vi "display AP status.vi"(7 "in or out display Refnum":refnum<vi>, 8 "error in":errorcluster={"status"=FALSE, "code"=-1950679034, "source"="Shared Variable in Large VAC READBACKS.vi<APPEND>\nThis error or warning occurred while reading the following Shared Variable:\n\\\\My Computer\\lowendshmc\\digital outputs\n\\\\192.168.1.200\\lowendshmc\\digital outputs"}, 9 "Aperture Status":T1, 10 "device control Refnum":refnum<vi>, 11 "use color control":bool) -> (0 "error out":errorcluster={"status"=FALSE, "code"=-1950679034, "source"="Shared Variable in Large VAC READBACKS.vi<APPEND>\nThis error or warning occurred while reading the following Shared Variable:\n\\\\My Computer\\lowendshmc\\digital outputs\n\\\\192.168.1.200\\lowendshmc\\digital outputs"})   [LabVIEW 2016, in "sub-VIs.lvlib"]
doc: "controls the display of if a cup or apt. is in the beamline"
uses:
  sub-VIs/sub-VIs.lvlib
  controls/Aperture states.ctl
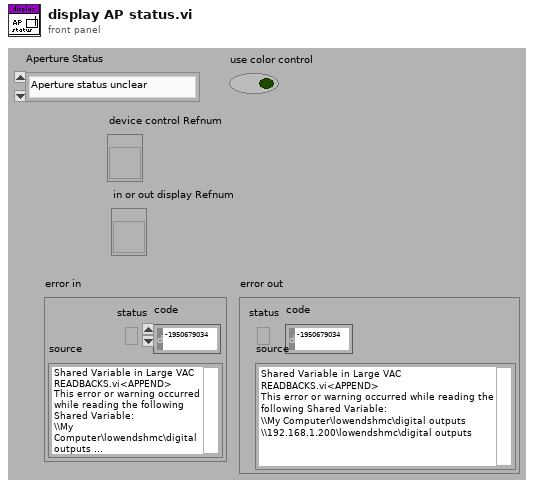
[diagram p1: front panel]
types:
  T1 = typedef "Aperture states.ctl" = enum16{"Aperture status unclear", "Aperture in", "Aperture out"}
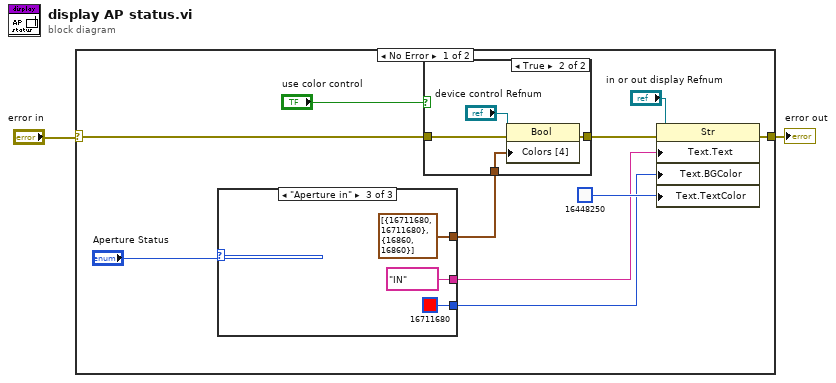
[diagram p0: block diagram]
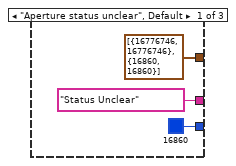
[diagram p3: hidden frame]
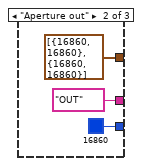
[diagram p4: hidden frame]
diagram:
  n1 = case shown="No Error" "error in" {
    selector: "error in" -> [w5 w27]
    tunnel: [w6 w27] -> w2
    frame No Error {
      n2 = case shown="\"Aperture in\"" "Aperture Status" {
        tunnel: ["Status Unclear" ("Text.Text") "OUT" ("Text.Text") "IN" ("Text.Text")] -> w9
        tunnel: [u32 16860 u32 16860 u32 16711680] -> w10
        tunnel: [cluster{u32, u32}[] [{16776746, 16776746}, {16860, 16860}] ("Colors [4]") cluster{u32, u32}[] [{16860, 16860}, {16860, 16860}] ("Colors [4]") cluster{u32, u32}[] [{16711680, 16711680}, {16860, 16860}] ("Colors [4]")] -> w12
        frame "Aperture status unclear", Default {
        }
        frame "Aperture out" {
        }
        frame "Aperture in" {
        }
      }
      n3 = case shown="True" "use color control" {
        tunnel: w12 -> [_ w17]
        tunnel: [w13 w16] -> w7
        tunnel: w5 -> [w13 w15]
        frame False {
        }
        frame True {
          n4 = property on="Property Node" class="Bool"(reference="device control Refnum", error in=w15, "Colors [4]"=w17) -> (error out=w16:errorcluster)  [unwired: 1 out]
        }
      }
      n5 = property on="Property Node" class="Str"(reference="in or out display Refnum", error in=w7, "Text.Text"=w9, "Text.BGColor"=w10, "Text.TextColor"=u32 16448250) -> (error out=w6:errorcluster)  [unwired: 1 out]
    }
    frame Error {
    }
  }
  "error out" <- w2
